vi "Process Image for Balls.vi"(0 "Src Image":T2, 1 "Color Mode 2":u16(ring)=2 items=["RGB", "HSL", "HSV", "HSI"], 9 "Color":T3, 11 "Area Cutoff %":dbl=0.4) -> (4 "Src Image Out":T2, 8 "First Threshold":T2, 10 "Fitted":T2, 15 "Potential":T1(array[cluster]))   [LabVIEW 2020]
doc: "Search image for circular colored particles. A second pass extracts a portion of the image, widens the color range, and fits a circle to the edge of the result."
uses:
  <vilib>/vision/Image Controls.llb/IMAQ Image.ctl
  <vilib>/vision/NI_Vision_Development_Module.lvlib
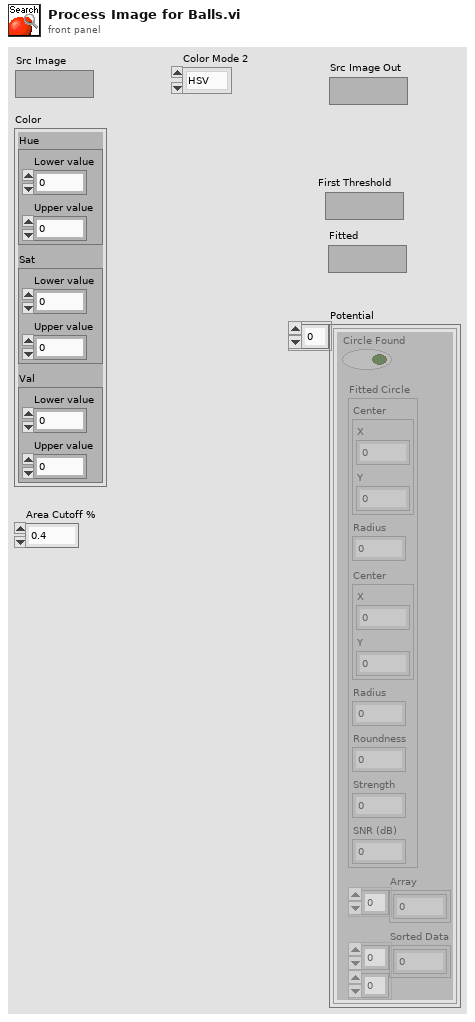
[diagram p1: front panel]
types:
  T1 = cluster{"Circle Found":bool, "Fitted Circle":cluster{"Center":cluster{"X":sgl, "Y":sgl}, "Radius":dbl, "Center":cluster{"X":sgl, "Y":sgl}, "Radius":dbl, "Roundness":dbl, "Strength":dbl, "SNR (dB)":dbl}, "Array":dbl[], "Sorted Data":dbl[][]}[]
  T2 = typedef "IMAQ Image.ctl" = refnum<image>
  T3 = cluster{"Hue ":cluster{"Lower value":i32, "Upper value":i32}, "Sat ":cluster{"Lower value":i32, "Upper value":i32}, "Val ":cluster{"Lower value":i32, "Upper value":i32}}
  T4 = typedef "Image Type" = u32
  T5 = typedef "Particle Parameters" = i32
  T6 = typedef "ROI Descriptor" = cluster{"Global Rectangle":i32[], "Contours":cluster{"ID":enum32{"External", "Internal"}, "Type":u32, "Coordinates":i32[]}[]}
  T7 = cluster{"Circle Found":bool, "Fitted Circle":cluster{"Center":cluster{"X":sgl, "Y":sgl}, "Radius":dbl, "Center":cluster{"X":sgl, "Y":sgl}, "Radius":dbl, "Roundness":dbl, "Strength":dbl, "SNR (dB)":dbl}, "Array":dbl[], "Sorted Data":dbl[][]}
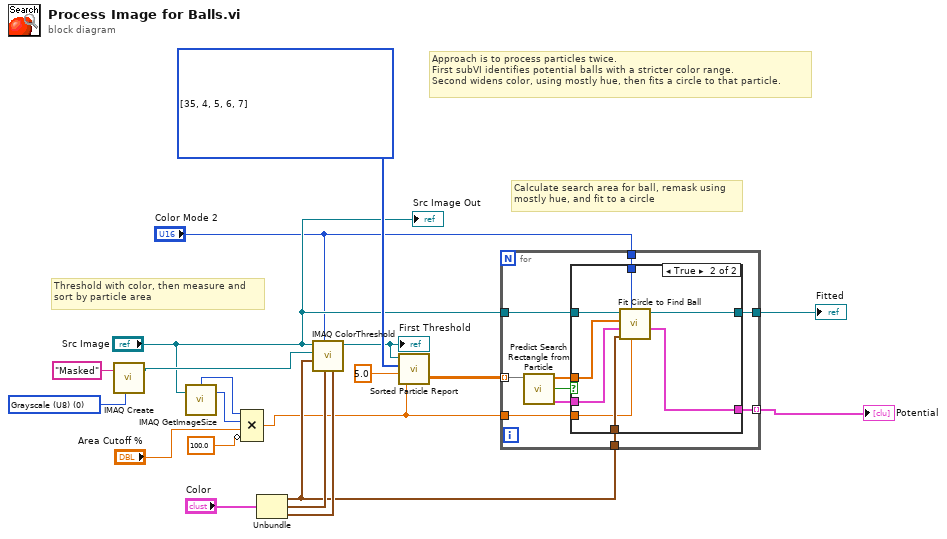
[diagram p0: block diagram]
diagram:
  w10 = T4 0 items=["Grayscale (U8)", "Grayscale (I16)", "Grayscale (SGL)", "Complex (CSG)", "RGB (U32)", "HSL (U32)", "RGB (U64)", "Grayscale (U16)"] ("Image Type")
  w19 = T5[] [35, 4, 5, 6, 7] items=["Center of Mass X", "Center of Mass Y", "First Pixel X", "First Pixel Y", "Bounding Rect Left", "Bounding Rect Top", "Bounding Rect Right", "Bounding Rect Bottom", "Max Feret Diameter Start X", "Max Feret Diameter Start Y", "Max Feret Diameter End X", "Max Feret Diameter End Y", "Max Horiz. Segment Length Left", "Max Horiz. Segment Length Right", "Max Horiz. Segment Length Row", "-", "Bounding Rect Width", "Bounding Rect Height", "Bounding Rect Diagonal", "Perimeter", "Convex Hull Perimeter", "Holes' Perimeter", "Max Feret Diameter", "Equivalent Ellipse Major Axis", "Equivalent Ellipse Minor Axis", "Equivalent Ellipse Minor Axis (Feret)", "Equivalent Rect Long Side", "Equivalent Rect Short Side", "Equivalent Rect Diagonal", "Equivalent Rect Short Side (Feret)", "Average Horiz. Segment Length", "Average Vert. Segment Length", "Hydraulic Radius", "Waddel Disk Diameter", "-", "Area", "Holes' Area", "Particle & Holes' Area", "Convex Hull Area", "Image Area", "-", "Number of Holes", "Number of Horiz. Segments", "Number of Vert. Segments", "-", "Orientation", "Max Feret Diameter Orientation", "-", "% Area/Image Area", "% Area/(Particle & Holes' Area)", "Ratio of Equivalent Ellipse Axes", "Ratio of Equivalent Rect Sides", "-", "Elongation Factor", "Compactness Factor", "Heywood Circularity Factor", "Type Factor", "-", "Sum X", "Sum Y", "Sum XX", "Sum XY", "Sum YY", "Sum XXX", "Sum XXY", "Sum XYY", "Sum YYY", "-", "Moment of Inertia XX", "Moment of Inertia XY", "Moment of Inertia YY", "Moment of Inertia XXX", "Moment of Inertia XXY", "Moment of Inertia XYY", "Moment of Inertia YYY", "Norm. Moment of Inertia XX", "Norm. Moment of Inertia XY", "Norm. Moment of Inertia YY", "Norm. Moment of Inertia XXX", "Norm. Moment of Inertia XXY", "Norm. Moment of Inertia XYY", "Norm. Moment of Inertia YYY", "Hu Moment 1", "Hu Moment 2", "Hu Moment 3", "Hu Moment 4", "Hu Moment 5", "Hu Moment 6", "Hu Moment 7"] ("Pixel Measurements")
  # "Approach is to process particles twice.\nFirst subVI identifies potential balls with a stricter color range.\nSecond widens color, using mostly hue, then fits a circle to that particle."
  # "Threshold with color, then measure and\nsort by particle area"
  # "Calculate search area for ball, remask using\nmostly hue, and fit to a circle"
  n1 = call "IMAQ Create"("Image Name"="Masked", "Image Type"=w10) -> ("New Image"=w8:T2)  [unwired: 3 in, 1 out]
  n2 = call "IMAQ GetImageSize"("Image"="Src Image") -> ("Y Resolution"=w5:i32, "X Resolution"=w6:i32)  [unwired: 3 in, 1 out]
  n3 = Compound Arithmetic op=MULTIPLY(w6, w5, "Area Cutoff %", invert 100.0 ("value")) -> (w3:dbl)
  n4 = Unbundle("Color") -> ("Hue"=w15:cluster{"Lower value":i32, "Upper value":i32}, "Sat"=w16:cluster{"Lower value":i32, "Upper value":i32}, "Val"=w17:cluster{"Lower value":i32, "Upper value":i32})
  n5 = call "IMAQ ColorThreshold"("Blue or Luma or Val or Inten Range"=w17, "Green or Sat Range"=w16, "Color Mode"="Color Mode 2", "Red or Hue Range"=w15, "Image Dst"=w8, "Image Src"="Src Image") -> ("Image Dst Out"=w14:T2)  [unwired: 4 in, 1 out]
  "First Threshold" <- w14
  n6 = call "Sorted Particle Report.vi"("Area Size Limit"=w3, "Particle Count Limit"=5.0, "Pixel Measurements"=w19, "Image in"=w14) -> ("Sorted Data"=w13:dbl[][])  [unwired: 1 out]
  n7 = for {
    tunnel: w13 -> [w30] mode=indexing
    tunnel: [w28] -> w11 mode=indexing
    tunnel: w15 -> [w26]
    tunnel: w3 -> [w23]
    tunnel: "Color Mode 2" -> [w24]
    tunnel: "Src Image" -> [w22]
    tunnel: [w21] -> w20
    n8 = call "Predict Search Rectangle from Particle.vi"("Sorted Data"=w30) -> ("ROI Descriptor"=w25:T6, "Valid"=w27:bool, "Rectangle ltrb"=w29:dbl[])  [unwired: 8 in]
    n9 = case shown="True" w27 {
      tunnel: w29 -> [_ w35]
      tunnel: [_ w39] -> w28
      tunnel: w22 -> [w31 w34]
      tunnel: w26 -> [_ w36]
      tunnel: w25 -> [_ w38]
      tunnel: w24 -> [_ w37]
      tunnel: w23 -> [_ w33]
      tunnel: [w31 w32] -> w21
      frame False {
      }
      frame True {
        n10 = call "Fit Circle to Find Ball.vi"("Area Size Limit"=w33, "Color Mode"=w37, "Hue"=w36, "ROI Descriptor"=w38, "Rectangle ltrb"=w35, "Color Image In"=w34) -> ("Potential Ball"=w39:T7, "Image out"=w32:T2)  [unwired: 4 in]
      }
    }
  }
  "Fitted" <- w20
  "Potential" <- w11
  "Src Image Out" <- "Src Image"
